vi "PI_GCS3_Configuration_Setup_Limits.vi"(0 "System no.":i32=1 min=1 step=1, 1 "Conn. Axes":string[](array[string]), 5 "error in":errorcluster) -> (14 "Positive Limit":dbl[](array[numeric]) format="%.6f", 16 "Negative Limit":dbl[](array[numeric]) format="%.6f", 19 "error out":errorcluster)   [LabVIEW 2020]
doc: "Gather positive and negative axes limits."
uses:
  ConfigurationMemoryType.ctl
panel:
  # "Gather positive and negative axes limits."
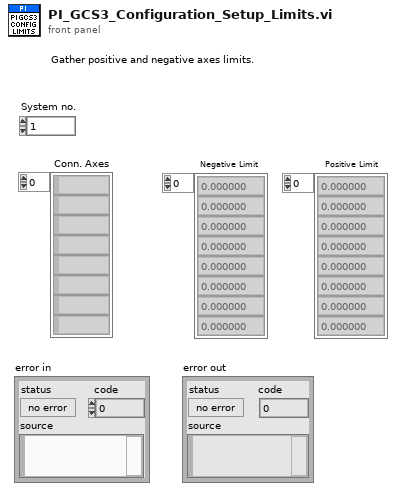
[diagram p1: front panel]
types:
  T1 = typedef "ConfigurationMemoryType.ctl" = enum16{"RAM", "TMP", "FLASH"}
  T2 = typedef "Parameter Set.ctl" = cluster{"Memory Type":T3, "Container Unit":string, "Function Unit":string, "Parameter ID":string, "Parameter Value":string}
  T3 = typedef "MemoryType.ctl" = enum16{"<No Setting>", "RAM", "FLASH", "TMP"}
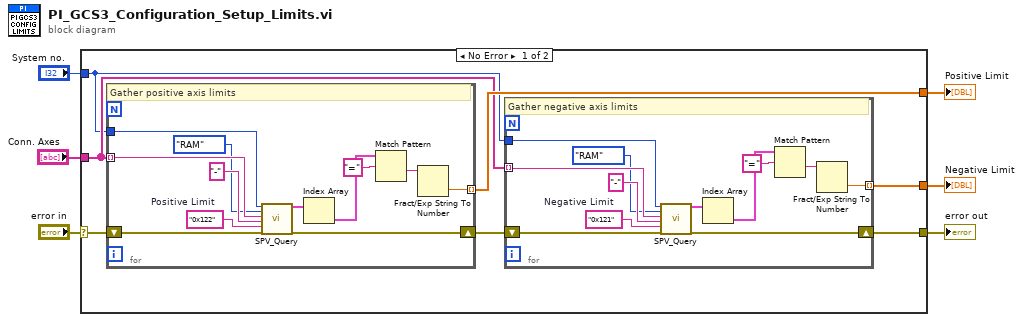
[diagram p0: block diagram]
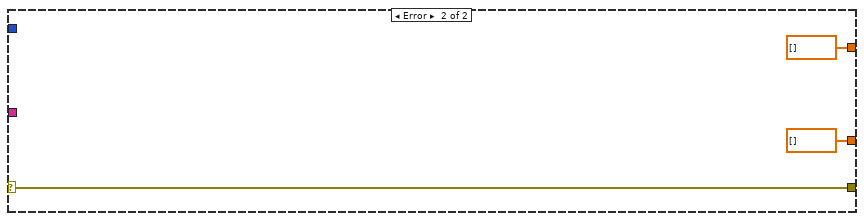
[diagram p2: hidden frame]
diagram:
  n1 = case shown="No Error" "error in" {
    selector: "error in" -> [w13 w40]
    tunnel: [w8 w40] -> w5
    tunnel: "Conn. Axes" -> [w10 _]
    tunnel: "System no." -> [w9 _]
    tunnel: [w7 dbl[] [] ("Negative Limit")] -> w2
    tunnel: [w12 dbl[] [] ("Negative Limit")] -> w1
    frame No Error {
      n2 = for {
        shift-right: [w37] -> w11
        shift-left: w13 -> [w31]
        tunnel: w9 -> [w33]
        tunnel: w10 -> [w35] mode=indexing
        tunnel: [w30] -> w12 mode=indexing
        w36 = "0x122"  # Positive Limit
        # "Gather positive axis limits"
        n3 = call "SPV_Query.vi"("System no."=w33, "Memory Type"=ConfigurationMemoryType."RAM" ("Target Memory Type"), "ContainerUnit"=w35, "FunctionUnit"="-", "ParameterID"=w36, "error in"=w31) -> ("Parameters"=w28:T2[], "error out"=w37:errorcluster)  [unwired: 12 in]
        n4 = Index Array(array=w28) -> (element=w27:T2)  [unwired: 1 in]
        n5 = Match Pattern(string=w27, regular expression="=") -> (after substring=w26:string)  [unwired: 1 in, 3 out]
        n6 = Fract/Exp String To Number(string=w26) -> (number=w30:dbl)  [unwired: 3 in, 1 out]
      }
      n7 = for {
        shift-right: [w19] -> w8
        shift-left: w11 -> [w24]
        tunnel: w9 -> [w20]
        tunnel: w10 -> [w22] mode=indexing
        tunnel: [w18] -> w7 mode=indexing
        w25 = "0x121"  # Negative Limit
        # "Gather negative axis limits"
        n8 = call "SPV_Query.vi"("System no."=w20, "Memory Type"=ConfigurationMemoryType."RAM" ("Target Memory Type"), "ContainerUnit"=w22, "FunctionUnit"="-", "ParameterID"=w25, "error in"=w24) -> ("Parameters"=w15:T2[], "error out"=w19:errorcluster)  [unwired: 12 in]
        n9 = Index Array(array=w15) -> (element=w16:T2)  [unwired: 1 in]
        n10 = Match Pattern(string=w16, regular expression="=") -> (after substring=w14:string)  [unwired: 1 in, 3 out]
        n11 = Fract/Exp String To Number(string=w14) -> (number=w18:dbl)  [unwired: 3 in, 1 out]
      }
    }
    frame Error {
    }
  }
  "error out" <- w5
  "Negative Limit" <- w2
  "Positive Limit" <- w1
